vi "Read Pct Encode.vi"(8 "error in (no error)":errorcluster, 11 "URI-Component in":refnum<class "URI-Component.lvclass">) -> (0 "error out":errorcluster, 2 "Pct Encode":bool, 3 "URI-Component out":refnum<class "URI-Component.lvclass">)   [LabVIEW 2013]
uses:
  URI-Component.lvclass
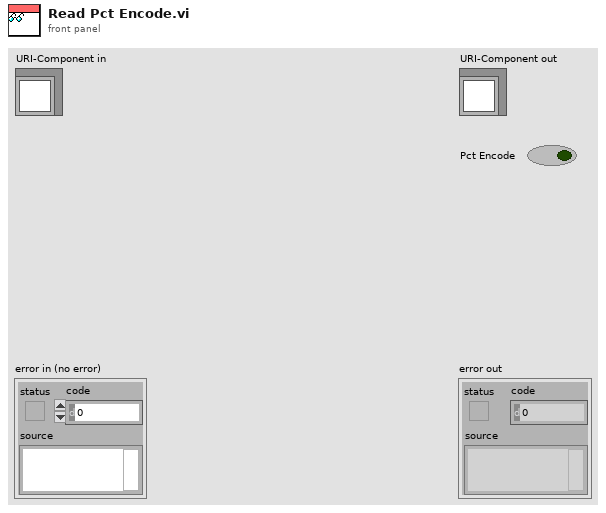
[diagram p1: front panel]
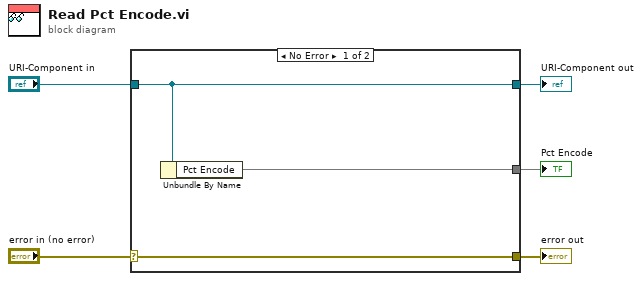
[diagram p0: block diagram]
diagram:
  n1 = case shown="No Error" "error in (no error)" {
    selector: "error in (no error)" -> [w8 w9]
    tunnel: [w8 w9] -> w4
    tunnel: [w7 w10] -> w2
    tunnel: "URI-Component in" -> [w7 w10]
    tunnel: [w6 _] -> w1
    frame No Error {
      n2 = Unbundle By Name(w7) -> ("Pct Encode"=w6)
    }
    frame Error {
    }
  }
  "error out" <- w4
  "URI-Component out" <- w2
  "Pct Encode" <- w1
